vi "Day1.2.vi"() -> ()   [LabVIEW 2023]
uses:
  <userlib>/_OpenG.lib/array/array.llb/Search 1D Array (I32)__ogtk.vi
  <userlib>/_OpenG.lib/array/array.llb/openg_array.lvlib
panel:
  out "Array":i32[](array[numeric])
  out "Sum":i32
  out "B":i32[](array[numeric])
  out "A":i32[](array[numeric])
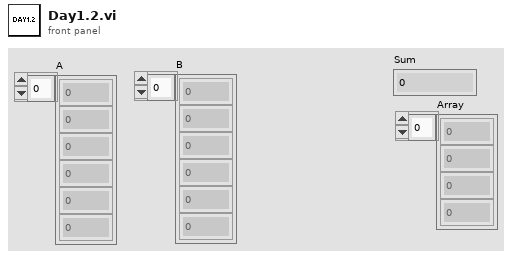
[diagram p1: front panel]
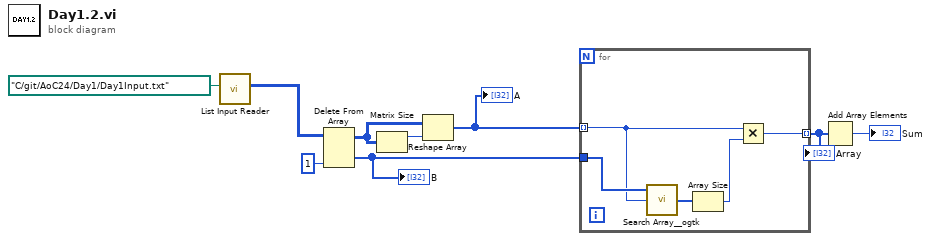
[diagram p0: block diagram]
diagram:
  n1 = call "List Input Reader.vi"("file path (dialog if empty)"=path "C:/git/AoC24/Day1/Day1Input.txt") -> ("Array"=w8:i32[][])  [unwired: 9 in, 1 out]
  n2 = Delete From Array(array=w8, index (col)=1 ("disabled index (col)")) -> (deleted portion=w4:i32[], array with subset deleted=w6:i32[][])  [unwired: 2 in]
  "B" <- w4
  n3 = Matrix Size(0:w6) -> (1:w5:i32)  [unwired: 1 out]
  n4 = Reshape Array(w6, w5) -> (w2:i32[])
  "A" <- w2
  n5 = for {
    tunnel: w2 -> [w10] mode=indexing
    tunnel: w4 -> [w14]
    tunnel: [w11] -> w1 mode=indexing
    n6 = call-poly <userlib>:"Search Array__ogtk.vi"("Array"=w14, "Element Data"=w10) -> ("Indices of Elements"=w12:i32[])  [unwired: 7 in]
    n7 = Array Size(array=w12) -> (size(s)=w13:i32)
    n8 = Multiply(x=w10, y=w13) -> (x*y=w11:i32)
  }
  "Array" <- w1
  n9 = Add Array Elements(numeric array=w1) -> (sum=→"Sum":i32)
